vi "Populate Tree with Categories.vi"(6 "Path & Icon":T1, 8 "error in":errorcluster, 11 "Tree Refnum in":refnum<vi>) -> (0 "error out":errorcluster, 3 "Tree Refnum out":refnum<vi>)   [LabVIEW 2020]
uses:
  Controls/Path&Icon.ctl
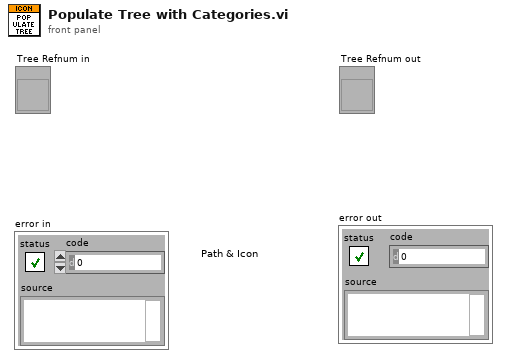
[diagram p1: front panel]
types:
  T1 = typedef "Path&Icon.ctl" = cluster{"Rectangle":cluster{"left":i16, "top":i16, "right":i16, "bottom":i16}, "Path":path, "Image":picture, "Filter":string, "FileName":string}
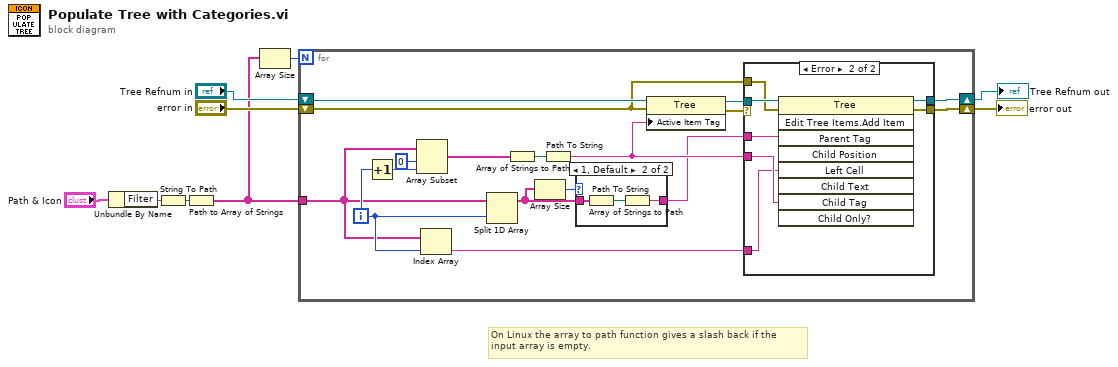
[diagram p0: block diagram]
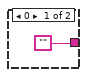
[diagram p2: hidden frame]
diagram:
  # "On Linux the array to path function gives a slash back if the \ninput array is empty."
  n1 = Unbundle By Name("Path & Icon") -> ("Filter"=w3:string)
  n2 = String To Path(string=w3) -> (path=w2:path)
  n3 = Path to Array of Strings(0:w2) -> (2:w1:string[])  [unwired: 1 out]
  n4 = Array Size(array=w1) -> (size(s)=w7:i32)
  n5 = for {
    N: w7 -> [_]
    tunnel: w1 -> [w18]
    shift-right: [w23] -> w6
    shift-left: "error in" -> [w16]
    shift-right: [w22] -> w5
    shift-left: "Tree Refnum in" -> [w26]
    i -> [w19]
    n6 = Increment(x=w19) -> (x+1=w21:i32)
    n7 = Array Subset(array=w18, index=0, length=w21) -> (w14:string[])
    n8 = Index Array(array=w18, index=w19) -> (element=w17:string)
    n9 = Split 1D Array(array=w18, index=w19) -> (first subarray=w11:string[])  [unwired: 1 out]
    n10 = Array of Strings to Path(0:w14) -> (2:w13:path)  [unwired: 1 out]
    n11 = Array Size(array=w11) -> (size(s)=w12:i32)
    n12 = Path To String(path=w13) -> (string=w15:string)
    n13 = case shown="1, Default" w12 {
      tunnel: w11 -> [_ w30]
      tunnel: ["" w28] -> w10
      frame 0 {
      }
      frame 1, Default {
        n14 = Array of Strings to Path(0:w30) -> (2:w29:path)  [unwired: 1 out]
        n15 = Path To String(path=w29) -> (string=w28:string)
      }
    }
    n16 = property class="Tree"(reference=w26, error in=w16, "Active Item Tag"=w15) -> (reference out=w24:refnum<vi>, error out=w25:errorcluster)
    n17 = case shown="Error" w25 {
      selector: w25 -> [w31 _]
      tunnel: w24 -> [w32 w39]
      tunnel: w10 -> [_ w38]
      tunnel: [w32 w37] -> w22
      tunnel: [w31 w36] -> w23
      tunnel: w15 -> [_ w35]
      tunnel: w17 -> [_ w34]
      tunnel: w16 -> [_ w33]
      frame No Error {
      }
      frame Error {
        n18 = invoke class="Tree" method="Edit Tree Items.Add Item"(reference=w39, error in=w33, "Parent Tag"=w38, "Left Cell"=w34, "Child Tag"=w35) -> (reference out=w37:refnum<vi>, error out=w36:errorcluster)  [unwired: 4 in, 7 out]
      }
    }
  }
  "error out" <- w6
  "Tree Refnum out" <- w5
